vi "Battery Scaling.vi"(8 "error in (no error)":errorcluster) -> (0 "error out":errorcluster, 3 "Battery_Scale":sgl)   [LabVIEW 2014]
uses:
  Battery_scale.vi
  <userlib>/UCSD Robotics Lab/Robotics-Cape/LV/libroboticscape.lvlib
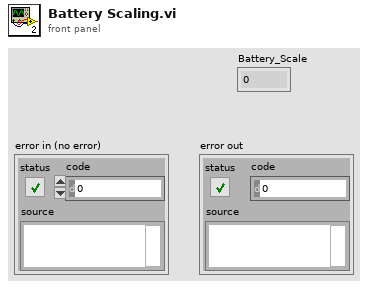
[diagram p1: front panel]
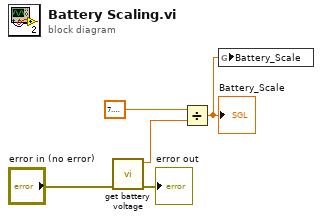
[diagram p0: block diagram]
diagram:
  n1 = call <userlib>:"get battery voltage.vi"("error in (no error)"="error in (no error)") -> ("error out"=→"error out":errorcluster, "function return"=w1:sgl)  [unwired: 9 in]
  n2 = Divide(x=sgl 7.4 ("y"), y=w1) -> (x/y=w3:sgl)
  "Battery_Scale" <- w3
  n3 = global write "Battery_scale.vi" "Battery_Scale"(w3) -> ()
